vi "GlobalInitialParamVals.vi"() -> ()   [LabVIEW 2015]
panel:
  in  "InitialParamVals":dbl[](array[numeric])
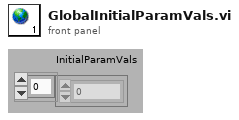
[diagram p1: front panel]
diagram:
